vi "Exercise 4.3 - Creating Local Variables.vi"() -> ()   [LabVIEW 2012]
panel:
  in  "stop":bool
  out "Boolean 3":bool
  out "Boolean 2":bool
  in  "Boolean":bool
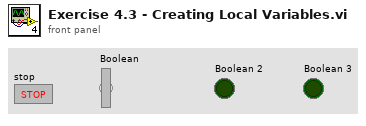
[diagram p1: front panel]
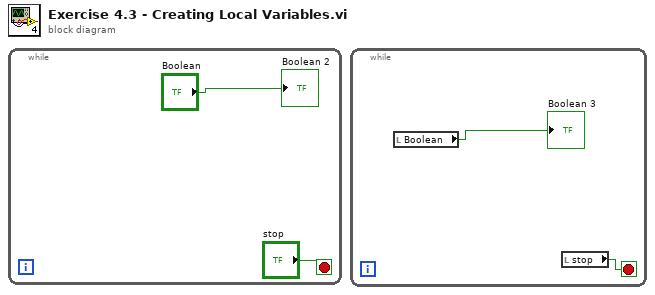
[diagram p0: block diagram]
diagram:
  n1 = while {
    stop <- "stop" stop-if-true
    "Boolean 2" <- "Boolean"
  }
  n2 = while {
    stop <- w4 stop-if-true
    n3 = local read "Boolean"() -> (→"Boolean 3":bool)
    n4 = local read "stop"() -> (w4:bool)
  }
